vi "logica de maquima.vi"() -> ()   [LabVIEW 2017]
uses:
  <vilib>/LabVIEW Interface for Arduino/Type Defs/Pin Mode.ctl
  <vilib>/LabVIEW Interface for Arduino/LabVIEW Interface for Arduino.lvlib
panel:
  in  "stop":bool
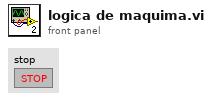
[diagram p1: front panel]
types:
  T1 = typedef "LabVIEW Interface for Arduino.lvlib/Arduino Resource.ctl" = cluster{"VISA resource":refnum<visa-resource-name>, "Board Type":T2, "Connection Type":enum8{"USB / Serial"}, "Bytes Per Packet (15)":u8}
  T2 = typedef "LabVIEW Interface for Arduino.lvlib/Board Type.ctl" = enum16{"Uno", "Dimuelanove w/Atmega 328", "Mega 2560"}
  T3 = typedef "LabVIEW Interface for Arduino.lvlib/Pin Mode.ctl" = enum8{"Input", "Output"}
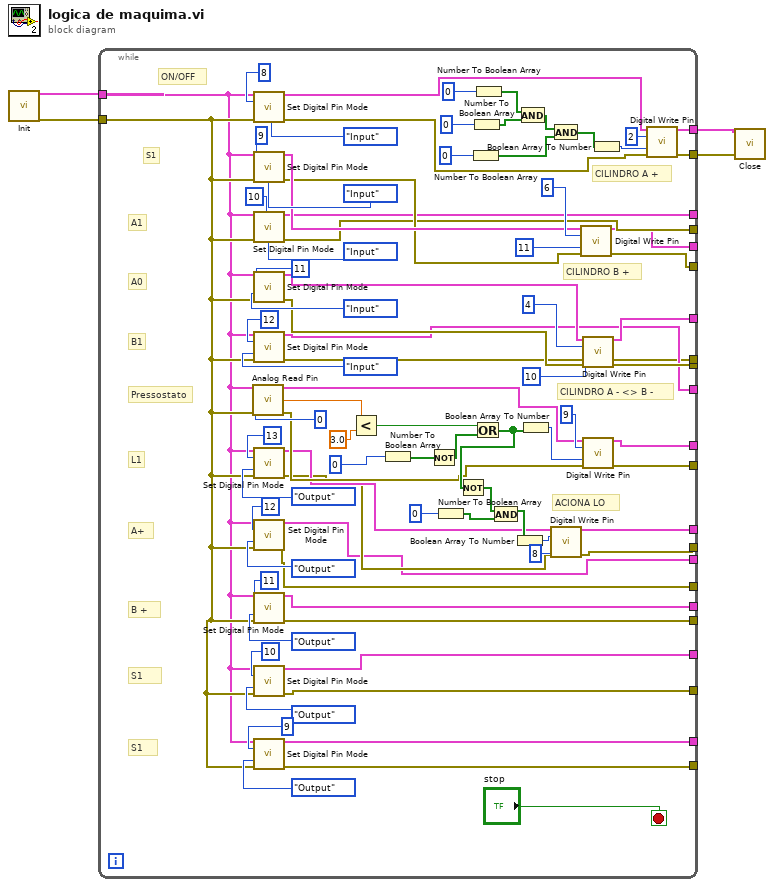
[diagram p0: block diagram]
diagram:
  n1 = call <vilib>:"Init.vi"() -> ("Arduino Resource"=w4:T1, "error out"=w3:errorcluster)  [unwired: 18 in]
  n2 = while {
    tunnel: w4 -> [w67]
    tunnel: w3 -> [w68]
    tunnel: [w35] -> _
    tunnel: [w34] -> _
    tunnel: [w31] -> w2
    tunnel: [w30] -> w1
    tunnel: [w29] -> _
    tunnel: [w28] -> _
    tunnel: [w27] -> _
    tunnel: [w26] -> _
    tunnel: [w25] -> _
    tunnel: [w21] -> _
    tunnel: [w18] -> _
    tunnel: [w17] -> _
    tunnel: [w14] -> _
    tunnel: [w13] -> _
    tunnel: [w12] -> _
    tunnel: [w11] -> _
    tunnel: [w10] -> _
    tunnel: [w9] -> _
    tunnel: [w8] -> _
    tunnel: [w7] -> _
    tunnel: [w6] -> _
    tunnel: [w5] -> _
    stop <- "stop" stop-if-true
    # "ACIONA LO"
    # "S1"
    # "S1"
    # "B +"
    # "A+"
    # "L1"
    # "Pressostato"
    # "B1"
    # "A1"
    # "A0"
    # "S1"
    # "ON/OFF"
    # "CILINDRO A - <> B -"
    # "CILINDRO B +"
    # "CILINDRO A +"
    n3 = call <vilib>:"Analog Read Pin.vi"("Arduino Resource"=w67, "Analog Input Pin (0)"=u8 0, "error in"=w68) -> ("Arduino Resource"=w20:T1, "Voltage"=w50:dbl, "error out"=w19:errorcluster)  [unwired: 10 in]
    n4 = call <vilib>:"Set Digital Pin Mode.vi"("Arduino Resource"=w67, "Digital I/O Pin"=u8 8, "Pin Mode (Input)"=Pin_Mode."Input", "error in"=w68) -> ("Arduino Resource"=w39:T1, "error out"=w38:errorcluster)  [unwired: 10 in]
    n5 = call <vilib>:"Set Digital Pin Mode.vi"("Arduino Resource"=w67, "Digital I/O Pin"=u8 9, "Pin Mode (Input)"=Pin_Mode."Input", "error in"=w68) -> ("Arduino Resource"=w37:T1, "error out"=w36:errorcluster)  [unwired: 10 in]
    n6 = call <vilib>:"Set Digital Pin Mode.vi"("Arduino Resource"=w67, "Digital I/O Pin"=u8 10, "Pin Mode (Input)"=Pin_Mode."Input", "error in"=w68) -> ("Arduino Resource"=w35:T1, "error out"=w34:errorcluster)  [unwired: 10 in]
    n7 = call <vilib>:"Set Digital Pin Mode.vi"("Arduino Resource"=w67, "Digital I/O Pin"=u8 11, "Pin Mode (Input)"=Pin_Mode."Input", "error in"=w68) -> ("Arduino Resource"=w33:T1, "error out"=w32:errorcluster)  [unwired: 10 in]
    n8 = call <vilib>:"Set Digital Pin Mode.vi"("Arduino Resource"=w67, "Digital I/O Pin"=u8 12, "Pin Mode (Input)"=Pin_Mode."Input", "error in"=w68) -> ("Arduino Resource"=w25:T1, "error out"=w21:errorcluster)  [unwired: 10 in]
    n9 = call <vilib>:"Set Digital Pin Mode.vi"("Arduino Resource"=w67, "Digital I/O Pin"=u8 13, "Pin Mode (Input)"=Pin_Mode."Output", "error in"=w68) -> ("Arduino Resource"=w16:T1, "error out"=w15:errorcluster)  [unwired: 10 in]
    n10 = call <vilib>:"Set Digital Pin Mode.vi"("Arduino Resource"=w67, "Digital I/O Pin"=u8 12, "Pin Mode (Input)"=Pin_Mode."Output", "error in"=w68) -> ("Arduino Resource"=w14:T1, "error out"=w13:errorcluster)  [unwired: 10 in]
    n11 = call <vilib>:"Set Digital Pin Mode.vi"("Arduino Resource"=w67, "Digital I/O Pin"=u8 11, "Pin Mode (Input)"=Pin_Mode."Output", "error in"=w68) -> ("Arduino Resource"=w10:T1, "error out"=w9:errorcluster)  [unwired: 10 in]
    n12 = call <vilib>:"Set Digital Pin Mode.vi"("Arduino Resource"=w67, "Digital I/O Pin"=u8 10, "Pin Mode (Input)"=Pin_Mode."Output", "error in"=w68) -> ("Arduino Resource"=w8:T1, "error out"=w7:errorcluster)  [unwired: 10 in]
    n13 = call <vilib>:"Set Digital Pin Mode.vi"("Arduino Resource"=w67, "Digital I/O Pin"=u8 9, "Pin Mode (Input)"=Pin_Mode."Output", "error in"=w68) -> ("Arduino Resource"=w6:T1, "error out"=w5:errorcluster)  [unwired: 10 in]
    n14 = Less?(x=w50, y=3.0) -> (x < y?=w47:bool)
    n15 = Number To Boolean Array(number=u32 0) -> (Boolean array=w48:bool[])
    n16 = Not(x=w48) -> (.not. x?=w46:bool[])
    n17 = Number To Boolean Array(number=u32 0) -> (Boolean array=w42:bool[])
    n18 = Number To Boolean Array(number=u32 0) -> (Boolean array=w61:bool[])
    n19 = Number To Boolean Array(number=u32 0) -> (Boolean array=w62:bool[])
    n20 = Or(x=w47, y=w46) -> (x .or. y?=w41:bool[])
    n21 = Not(x=w41) -> (.not. x?=w43:bool[])
    n22 = Number To Boolean Array(number=u32 0) -> (Boolean array=w63:bool[])
    n23 = And(x=w43, y=w42) -> (x .and. y?=w23:bool[])
    n24 = Boolean Array To Number(Boolean array=w23) -> (number=w24:u32)
    n25 = And(x=w63, y=w62) -> (x .and. y?=w60:bool[])
    n26 = Boolean Array To Number(Boolean array=w41) -> (number=w44:u32)
    n27 = And(x=w60, y=w61) -> (x .and. y?=w59:bool[])
    n28 = call <vilib>:"Digital Write Pin.vi"("Arduino Resource"=w16, "Digital I/O Pin (0)"=w24, "Value (0)"=u8 8, "error in"=w15) -> ("Arduino Resource"=w12:T1, "error out"=w11:errorcluster)  [unwired: 10 in]
    n29 = call <vilib>:"Digital Write Pin.vi"("Arduino Resource"=w37, "Digital I/O Pin (0)"=u8 6, "Value (0)"=u8 11, "error in"=w36) -> ("Arduino Resource"=w29:T1, "error out"=w28:errorcluster)  [unwired: 10 in]
    n30 = call <vilib>:"Digital Write Pin.vi"("Arduino Resource"=w33, "Digital I/O Pin (0)"=u8 4, "Value (0)"=u8 10, "error in"=w32) -> ("Arduino Resource"=w27:T1, "error out"=w26:errorcluster)  [unwired: 10 in]
    n31 = call <vilib>:"Digital Write Pin.vi"("Arduino Resource"=w20, "Digital I/O Pin (0)"=u8 9, "Value (0)"=w44, "error in"=w19) -> ("Arduino Resource"=w18:T1, "error out"=w17:errorcluster)  [unwired: 10 in]
    n32 = Boolean Array To Number(Boolean array=w59) -> (number=w58:u32)
    n33 = call <vilib>:"Digital Write Pin.vi"("Arduino Resource"=w39, "Digital I/O Pin (0)"=u8 2, "Value (0)"=w58, "error in"=w38) -> ("Arduino Resource"=w31:T1, "error out"=w30:errorcluster)  [unwired: 10 in]
  }
  n34 = call <vilib>:"Close.vi"("Arduino Resource"=w2, "error in"=w1) -> ()  [unwired: 13 in, 1 out]
